vi "25-Host Accepts Off-Line.vi"(8 "error in":errorcluster, 11 "Off-Line":bool) -> (0 "error out":errorcluster)   [LabVIEW 2020, in "SECS Scenarios.lvlib" / "Scenarios Class.lvclass"]
uses:
  Scenarios Class.lvclass
  25-Host Accepts Off-Line.ctl
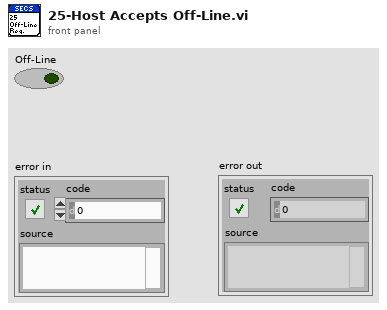
[diagram p1: front panel]
types:
  T1 = typedef "SECS Scenarios.lvlib/Scenarios Class.lvclass/25-Host Accepts Off-Line.ctl" = cluster{"Off-Line":bool}
  T2 = typedef "SECS Scenarios.lvlib/Scenarios Class.lvclass/Request Refnum.ctl" = cluster{"11-Alarm Management":refnum<user-event>, "07-Event Report From Equipment":refnum<user-event>, "14-Process Program Creating Editing or Deleting":refnum<user-event>, "21-Material Movement":refnum<user-event>, "23-Equipment Sends Information to Host":refnum<user-event>, "24-Host Accepts On-Line Request from Equipment":refnum<user-event>, "25-Host Refuses On-Line Request":refnum<user-event>, "29-Equipment Requests Time Value from Host":refnum<user-event>, "33-Update Trace Data":refnum<user-event>}
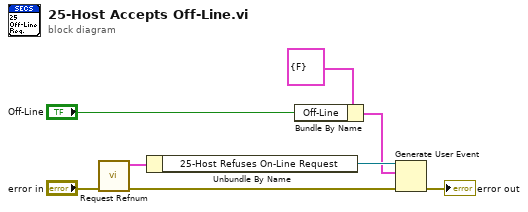
[diagram p0: block diagram]
diagram:
  n1 = call "Request Refnum.vi"("error in"="error in") -> ("error out"=w6:errorcluster, "Request Refnum"=w7:T2)  [unwired: 9 in]
  n2 = Unbundle By Name(w7) -> ("25-Host Refuses On-Line Request"=w5:refnum<user-event>)
  n3 = Bundle By Name(cluster=T1 {"Off-Line"=FALSE} ("25-Host Refuses On-Line Request"), "Off-Line"="Off-Line") -> (w4:T1)
  n4 = Generate User Event(user event=w5, event data cluster=w4, error in=w6) -> (error out=→"error out":errorcluster)  [unwired: 1 in, 1 out]
